vi "IsRunning.vi"(11 "JQMHModule in":refnum<class "Module.lvclass">) -> (2 "Is Running?":bool, 3 "JQMHModule out":refnum<class "Module.lvclass">)   [LabVIEW 2024, in "Module.lvclass"]
uses:
  Module.lvclass
  Module.lvclass/Module.ctl
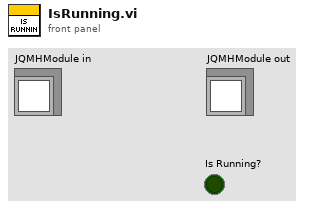
[diagram p1: front panel]
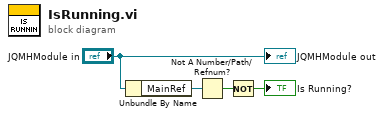
[diagram p0: block diagram]
diagram:
  n1 = Unbundle By Name("JQMHModule in") -> ("MainRef"=w3:refnum<vi>)
  n2 = Not A Number/Path/Refnum?(number/path/refnum=w3) -> (NaN/Path/Refnum?=w2:bool)
  n3 = Not(x=w2) -> (.not. x?=→"Is Running?":bool)
  "JQMHModule out" <- "JQMHModule in"
